vi "Get Car Wash Option Started Event.vi"(11 "Car Wash Option Started in":refnum<class "Car Wash Option Started.lvclass">) -> (1 "Name":string, 3 "Option":string)   [LabVIEW 2016, in "CLD Exam - Car Wash.lvlib" / "Car Wash Option Started.lvclass"]
uses:
  Car Wash Option Started.lvclass
  D:/Repos/Stream/software/Mediator/Classes/Message Interface/Message Interface.lvclass
  Car Wash Option Started.lvclass/Car Wash Option Started.ctl
  Mediator/Classes/Message Interface/Message Interface.lvclass
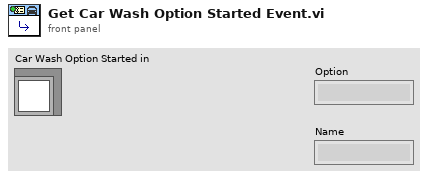
[diagram p1: front panel]
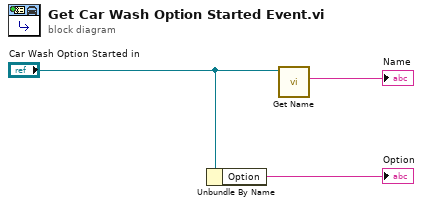
[diagram p0: block diagram]
diagram:
  n1 = Unbundle By Name("Car Wash Option Started in") -> ("Option"=→"Option":string)
  n2 = call "Get Name.vi"("Message Interface in"="Car Wash Option Started in") -> ("Name"=→"Name":string)  [unwired: 8 in, 2 out]
